vi "Update Status.vi"(8 "error in (no error)":errorcluster, 10 "Status":string, 11 "Execution UI In":refnum<class "Execution UI V2.lvclass">) -> (0 "error out":errorcluster, 3 "Execution UI Out":refnum<class "Execution UI V2.lvclass">)   [LabVIEW 2020, in "Execution UI V2.lvclass"]
uses:
  Execution UI V2.lvclass
  C:/Git/astemes-lunit/source/Application Framework/Process Classes/Process/Process.lvclass
  Application Framework/Process Classes/Process/Process.lvclass/Process.ctl
  Execution UI V2.lvclass/Execution UI V2.ctl
  Application Framework/Process Classes/Process/Process.lvclass
  C:/Git/astemes-lunit/source/Rewrite Project/Execution UI/Execution UI V2.lvclass
  C:/Git/astemes-lunit/source/Rewrite Project/Result Observer/Result Observer.lvclass
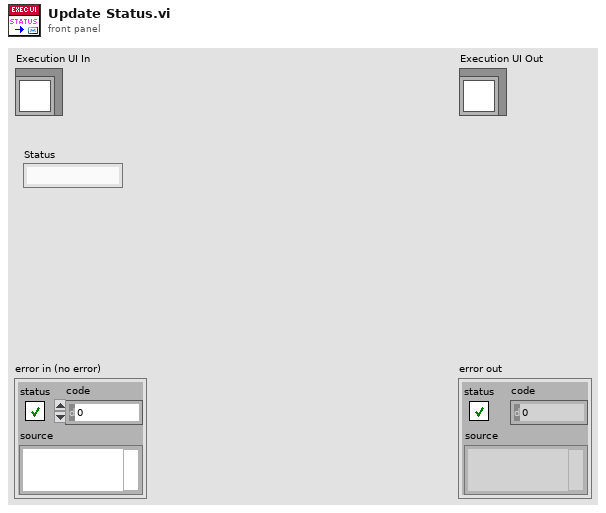
[diagram p1: front panel]
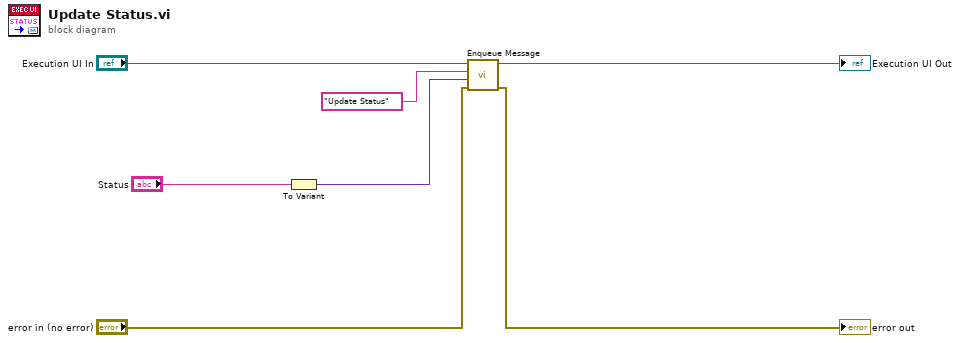
[diagram p0: block diagram]
diagram:
  n1 = To Variant(anything="Status") -> (Variant=w3:variant)
  n2 = call "Enqueue Message.vi"("error in (no error)"="error in (no error)", "Message Data"=w3, "Message"="Update Status", "Process In"="Execution UI In") -> ("error out"=→"error out":errorcluster, "Process Out"=→"Execution UI Out":refnum<class "Execution UI V2.lvclass">)  [unwired: 6 in]
